vi "ADQ214 Register Name Lookup.vi"(7 "address":u32, 8 "error in (no error)":errorcluster, 9 "rn":string, 10 "adq214_num":i32, 11 "adq_cu_ptr":u32) -> (0 "error out":errorcluster, 2 "function return":u32, 3 "adq_cu_ptr out":u32, 5 "address out":u32)   [LabVIEW 8.6, in "ADQAPI.lvlib"]
doc: "extern \"C\" __declspec(dllimport) unsigned int ADQ214_RegisterNameLookup(void* adq_cu_ptr, int adq214_num, const char* rn, unsigned int* address);"
uses:
  ADQAPI.lvlib
  F:/HRT/Sp Devices Thesis/ADQ-214 project (H R)/ADQAPI.dll
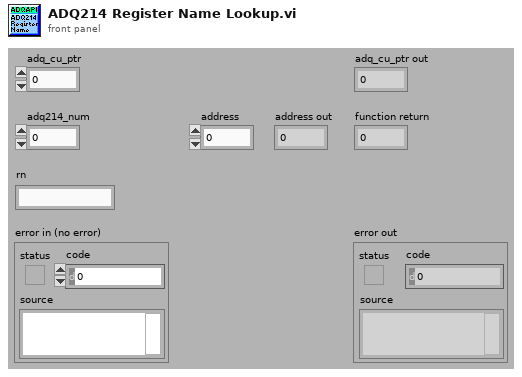
[diagram p1: front panel]
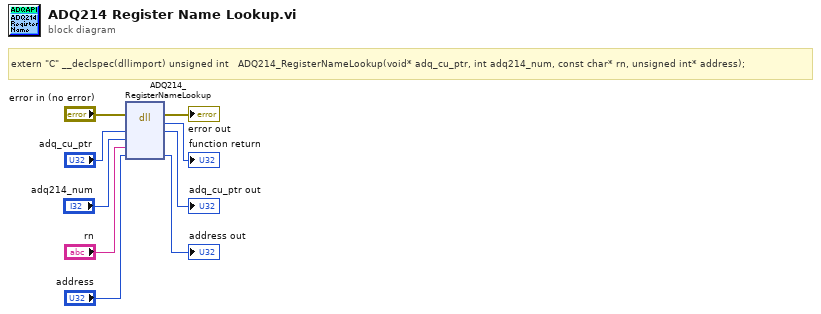
[diagram p0: block diagram]
diagram:
  # "extern \"C\" __declspec(dllimport) unsigned int   ADQ214_RegisterNameLookup(void* adq_cu_ptr, int adq214_num, const char* rn, unsigned int* address);"
  n1 = dll-call lib="F:/HRT/Sp Devices Thesis/ADQ-214 project (H R)/ADQAPI.*" fn="ADQ214_RegisterNameLookup"(error in="error in (no error)", "adq_cu_ptr"="adq_cu_ptr", "adq214_num"="adq214_num", "rn"="rn", "address"="address") -> (error out=→"error out":errorcluster, →"function return":u32, "adq_cu_ptr"=→"adq_cu_ptr out":u32, "address"=→"address out":u32)  [unwired: 4 in, 1 out]
